vi "Do.vi"(8 "error in (no error)":errorcluster, 10 "Actor in":refnum<class "Actor.lvclass">, 11 "Send Software Hold Trigger [HT] Msg":refnum<class "Send Software Hold Trigger [HT] Msg.lvclass">) -> (0 "error out":errorcluster, 2 "Actor out":refnum<class "Actor.lvclass">)   [LabVIEW 2014, in "CS++Fgen.lvlib" / "Send Software Hold Trigger [HT] Msg.lvclass"]
doc: "This VI delivers the message to the actor by calling the appropriate method(s) on the actor."
uses:
  Send Software Hold Trigger [HT] Msg.lvclass
  <vilib>/ActorFramework/Actor/Actor.lvclass
  CS++Fgen/CS++Fgen.lvclass
  CSPP_Core/Actors/CS++PVMonitor Messages/CS++PVUpdate Msg/CS++PVUpdate Msg.lvclass/CS++PVUpdate Msg.ctl
  CSPP_Core/Classes/CS++ProcessVariables/ProcessVariable/PV.lvclass/PV.ctl
  Send Software Hold Trigger [HT] Msg.lvclass/Send Software Hold Trigger [HT] Msg.ctl
  CSPP_Core/Classes/CS++ProcessVariables/ProcessVariable/PV.lvclass
  CSPP_Core/Actors/CS++PVMonitor Messages/CS++PVUpdate Msg/CS++PVUpdate Msg.lvclass
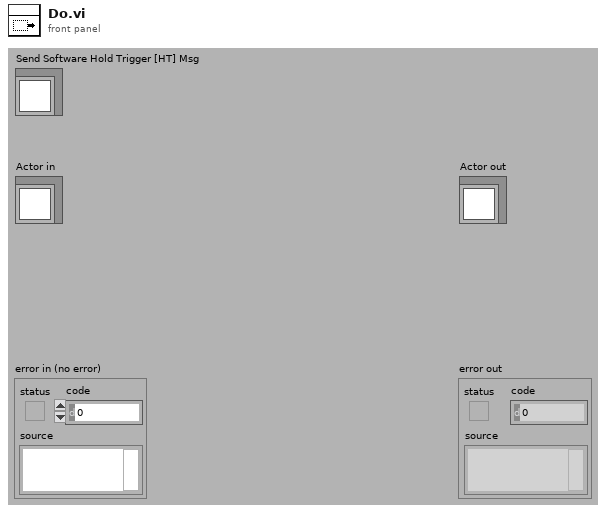
[diagram p1: front panel]
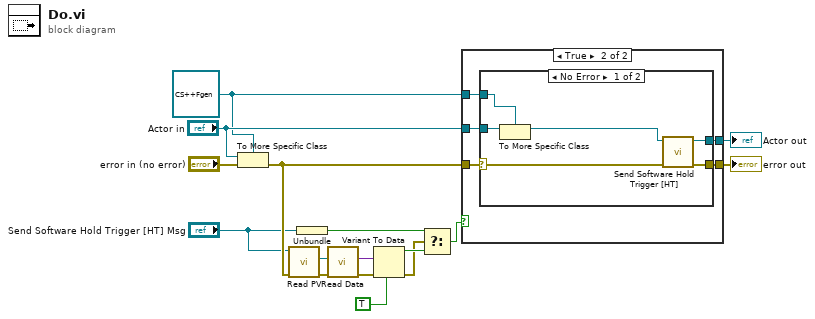
[diagram p0: block diagram]
diagram:
  w12 = refnum<class "CS++Fgen.lvclass"> refnum ("Actor in")
  n1 = To More Specific Class(target class=w12, reference="Actor in", error in="error in (no error)") -> (error out=w3:errorcluster)  [unwired: 1 out]
  n2 = call "Read PV.vi"("error in (no error)"=w3, "CS++PVUpdate Msg in"="Send Software Hold Trigger [HT] Msg") -> ("error out"=w5:errorcluster, "PV"=w11:refnum<class "PV.lvclass">)  [unwired: 7 in, 1 out]
  n3 = Unbundle("Send Software Hold Trigger [HT] Msg") -> (w8:bool)
  n4 = call "Read Data.vi"("error in (no error)"=w5, "PV in"=w11) -> ("error out"=w6:errorcluster, "Data"=w9:variant)  [unwired: 7 in, 1 out]
  n5 = Variant To Data(error in=w6, type=TRUE, Variant=w9) -> (data=w10:bool, error out=w7:errorcluster)
  n6 = Select(t=w8, s=w7, f=w10) -> (s? t:f=w1:bool)
  n7 = case shown="True" w1 {
    tunnel: [w17 w23] -> w15
    tunnel: [w18 w22] -> w14
    tunnel: "Actor in" -> [w18 w21]
    tunnel: w12 -> [_ w20]
    tunnel: w3 -> [w17 w19]
    frame False {
    }
    frame True {
      n8 = case shown="No Error" w19 {
        selector: w19 -> [w27 w31]
        tunnel: [w29 w31] -> w23
        tunnel: [w28 w30] -> w22
        tunnel: w21 -> [w26 w30]
        tunnel: w20 -> [w25 _]
        frame No Error {
          n9 = To More Specific Class(target class=w25, reference=w26) -> (specific class reference=w24:refnum<class "CS++Fgen.lvclass">)  [unwired: 1 in, 1 out]
          n10 = call "Send Software Hold Trigger [HT].vi"("error in (no error)"=w27, "CS++Fgen in"=w24) -> ("error out"=w29:errorcluster, "CS++Fgen out"=w28:refnum<class "CS++Fgen.lvclass">)  [unwired: 8 in]
        }
        frame Error {
          # "If type check fails, pass the original object out again."
        }
      }
    }
  }
  "error out" <- w15
  "Actor out" <- w14
